vi "Status.vi"(8 "error in (no error)":errorcluster, 11 "Sonicator Module State Cluster":T1={"State"=enum."Idle", "Start Time"=timestamp(0 s since 1904-01-01), "Current Time"=timestamp(0 s since 1904-01-01), "Sonicator Module Config"={"GUID"="", "Drop Coords"={"Horizontal"=0, "Vertical"=0}, "Process Name"="", "User name"="", "Queue Name"="", "Settings"={"Cycle Period"=500.0, "Sonicator Type"="Sonic Systems P100", "SS P100 Settings"={"VISA resource name"="", "Simulated?"=FALSE}, "Setpoint (µm)"=0.0, "Cutoff (W)"=0.0}, "Load Count"=0}, "Output Error"=FALSE, "Log Started"=FALSE, "First Iteration"=FALSE, "Data"={"Sonicator Amp Value"=0.0, "Sonicator Power Value"=0.0}, "Sonicator On?"=enum."Off"}) -> (0 "error out":errorcluster, 3 "Sonicator Module State Cluster":T1={"State"=enum."Idle", "Start Time"=timestamp(0 s since 1904-01-01), "Current Time"=timestamp(0 s since 1904-01-01), "Sonicator Module Config"={"GUID"="", "Drop Coords"={"Horizontal"=0, "Vertical"=0}, "Process Name"="", "User name"="", "Queue Name"="", "Settings"={"Cycle Period"=500.0, "Sonicator Type"="Sonic Systems P100", "SS P100 Settings"={"VISA resource name"="", "Simulated?"=FALSE}, "Setpoint (µm)"=0.0, "Cutoff (W)"=0.0}, "Load Count"=0}, "Output Error"=FALSE, "Log Started"=FALSE, "First Iteration"=FALSE, "Data"={"Sonicator Amp Value"=0.0, "Sonicator Power Value"=0.0}, "Sonicator On?"=enum."Off"})   [LabVIEW 2018, in "Sonicator Module.lvlib" / "Sonicator Module Engine.lvlib"]
uses:
  Sonicator Module Engine.lvlib
  Feed Module/Controls/Sonicator Module State Cluster.ctl
  Pump Module Folder/Measure Instrument/State Enum.ctl
  Feed Module/Controls/Sonicator Module Config Cluster.ctl
  <vilib>/Utility/miscctls.llb/LVPoint32TypeDef.ctl
  Feed Module/Controls/Sonicator Module Settings Cluster.ctl
  Sonic Systems P100/Sonic Systems P100 Settings.ctl
  Tag VIs/Tag FGV Operation Enum.ctl
  Shared Variables/Dynamic Shared Variables.lvlib
  Sonic Systems P100/Sonic Systems P100.lvlib
  Pump Module Folder/Measure Instrument/Pump Module Engine.lvlib
  Sonicator Module.lvlib
panel:
  # "Sonicator Settings"
  # "Sonicator Settings"
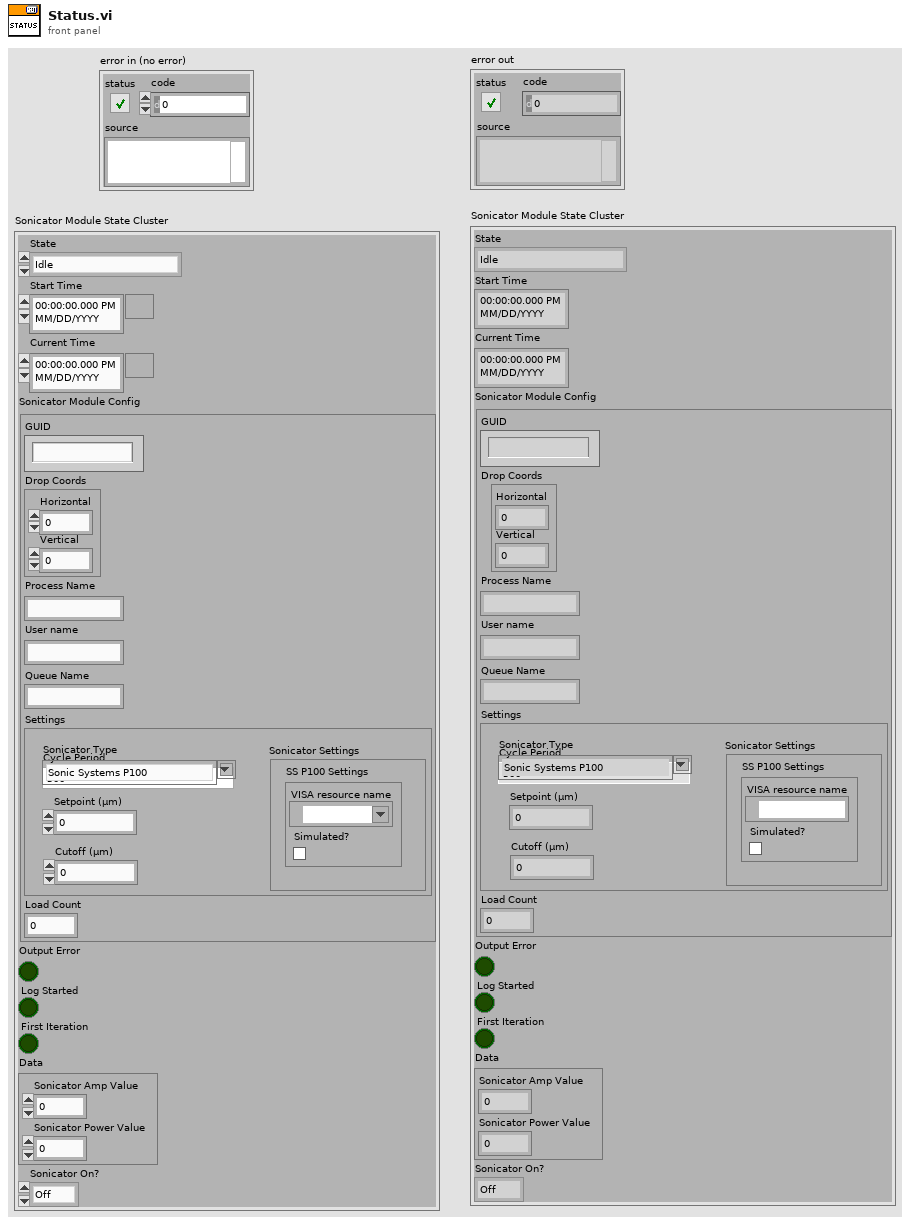
[diagram p1: front panel]
types:
  T1 = typedef "Sonicator Module.lvlib/Sonicator Module State Cluster.ctl" = cluster{"State":T2, "Start Time":timestamp, "Current Time":timestamp, "Sonicator Module Config":T3, "Output Error":bool, "Log Started":bool, "First Iteration":bool, "Data":cluster{"Sonicator Amp Value":dbl, "Sonicator Power Value":dbl}, "Sonicator On?":enum16{"Off", "On", "Not Initialized", "Over Cutoff"}}
  T2 = typedef "Pump Module.lvlib/Pump Module Engine.lvlib/State Enum.ctl" = enum16{"Measuring", "Idle", "Paused"}
  T3 = typedef "Sonicator Module.lvlib/Sonicator Module Config Cluster.ctl" = cluster{"GUID":string, "Drop Coords":T4, "Process Name":string, "User name":string, "Queue Name":string, "Settings":T5, "Load Count":i32}
  T4 = typedef "LVPoint32TypeDef.ctl" = cluster{"Horizontal":i32, "Vertical":i32}
  T5 = typedef "Sonicator Module.lvlib/Sonicator Module Settings Cluster.ctl" = cluster{"Cycle Period":dbl, "Sonicator Type":string, "SS P100 Settings":T6, "Setpoint (µm)":dbl, "Cutoff (W)":dbl}
  T6 = typedef "Sonic Systems P100.lvlib/Sonic Systems P100 Settings.ctl" = cluster{"VISA resource name":refnum<visa-resource-name>, "Simulated?":bool}
  T7 = typedef "Tag FGV Operation Enum.ctl" = enum16{"Init", "Set Notification Queue", "Create Tag", "Commit", "Write Tag (Numeric)", "Write Tag (Boolean)", "Read All Tags", "Read One Tag", "Delete Tag Category", "Set Alarm Parameters (Numeric)", "Set Alarm Parameters (Boolean)", "Enable All Alarms", "Disable All Alarms", "Delete All Tags", "Read Alarms", "Ack Alarm", "Read Alarm Parameters (Numeric)", "Read Alarm Parameters (Boolean)"}
  T8 = cluster{"Amplitude Tag":string, "Power Tag":string, "Output Device Tag":string}
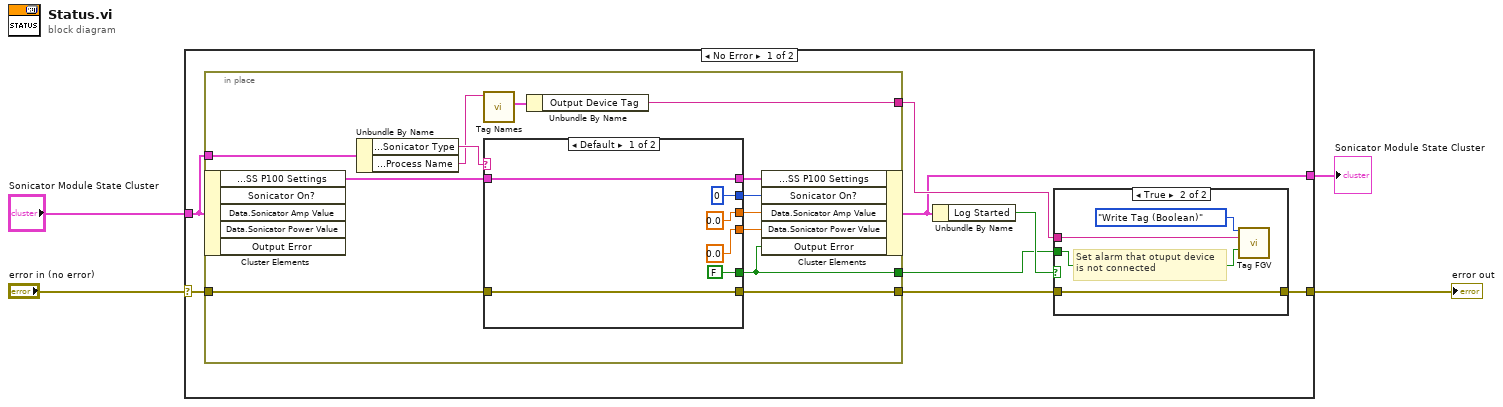
[diagram p0: block diagram]
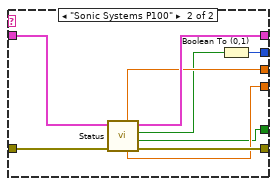
[diagram p2: hidden frame]
diagram:
  n1 = case shown="No Error" "error in (no error)" {
    selector: "error in (no error)" -> [w12 w47]
    tunnel: [w9 w47] -> w3
    tunnel: "Sonicator Module State Cluster" -> [w6 w46]
    tunnel: [w5 w46] -> w1
    frame No Error {
      n2 = in-place {
        in-place-border: w12 -> [w19]
        in-place-border: [w25] -> w11
        in-place-border: [w20] -> w10
        in-place-border: w6 -> [w15]
        in-place-border: [w16] -> w7
        n3 = in-place-cluster #1(w6) -> ("Sonicator Module Config.Settings.SS P100 Settings"=w22:T6)  [unwired: 4 out]
        n4 = Unbundle By Name(w15) -> ("Sonicator Module Config.Settings.Sonicator Type"=w23:string, "Sonicator Module Config.Process Name"=w14:string)
        n5 = call "Tag Names.vi"("Process Name"=w14) -> ("SC Tags"=w24:T8)  [unwired: 8 in, 2 out]
        n6 = case shown="Default" w23 {
          tunnel: w22 -> [w31 w40]
          tunnel: [w31 w39] -> w21
          tunnel: [w27 w38] -> w20
          tunnel: w19 -> [w27 w37]
          tunnel: [0.0 ("Amplitude") w36] -> w18
          tunnel: [0.0 ("Power") w35] -> w17
          tunnel: [FALSE ("Connection Error") w34] -> w16
          tunnel: [i16 0 w33] -> w13
          frame Default {
          }
          frame "Sonic Systems P100" {
            n7 = call "Status.vi"("error in (no error)"=w37, "SS P100 Settings In"=w40) -> ("error out"=w38:errorcluster, "Connection Error"=w34:bool, "Running"=w32:bool, "SS P100 Settings Out"=w39:T6, "Power"=w35:dbl, "Amplitude"=w36:dbl)  [unwired: 4 in]
            n8 = Boolean To (0,1)(Boolean=w32) -> (0, 1=w33:i16)
          }
        }
        n9 = Unbundle By Name(w24) -> ("Output Device Tag"=w25:string)
        n10 = in-place-cluster #1("Sonicator Module Config.Settings.SS P100 Settings"=w21, "Sonicator On?"=w13, "Data.Sonicator Amp Value"=w18, "Data.Sonicator Power Value"=w17, "Output Error"=w16) -> (w5:T1)
      }
      n11 = Unbundle By Name(w5) -> ("Log Started"=w8:bool)
      n12 = case shown="True" w8 {
        tunnel: w11 -> [_ w45]
        tunnel: w10 -> [w41 w44]
        tunnel: [w41 w44] -> w9
        tunnel: w7 -> [_ w42]
        frame False {
        }
        frame True {
          # "Set alarm that otuput device\nis not connected"
          n13 = call "Tag FGV.vi"("Operation"=Tag_FGV_Operation_Enum."Write Tag (Boolean)", "Tag Name"=w45, "Data"=w42) -> ()  [unwired: 5 in, 8 out]
        }
      }
    }
    frame Error {
    }
  }
  "error out" <- w3
  "Sonicator Module State Cluster" <- w1
